vi "Get Literal Value.vi"(11 "Array In":bool[](array[boolean])) -> (2 "Number":u64, 3 "Array Out":bool[](array[boolean]))   [LabVIEW 2021]
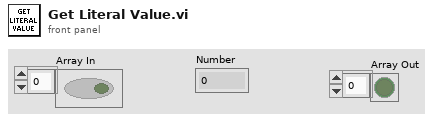
[diagram p1: front panel]
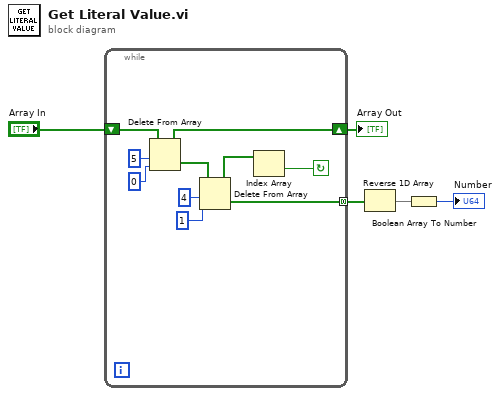
[diagram p0: block diagram]
diagram:
  n1 = while {
    shift-right: [w14] -> w1
    shift-left: "Array In" -> [w15]
    tunnel: [w8] -> w4 mode=concatenating
    stop <- w6 continue-if-true
    n2 = Delete From Array(array=w15, length=5, index=0) -> (deleted portion=w11:bool[], array with subset deleted=w14:bool[])
    n3 = Delete From Array(array=w11, length=4, index=1) -> (deleted portion=w8:bool[], array with subset deleted=w7:bool[])
    n4 = Index Array(array=w7) -> (element=w6:bool)  [unwired: 1 in]
  }
  "Array Out" <- w1
  n5 = Reverse 1D Array(array=w4) -> (reversed array=w3:bool[])
  n6 = Boolean Array To Number(Boolean array=w3) -> (number=→"Number":u64)
